vi "Logging Active.vi"(8 "error in (no error)":errorcluster, 11 "Active in":refnum<class "Active.lvclass">) -> (0 "error out":errorcluster, 3 "Active out":refnum<class "Active.lvclass">)   [LabVIEW 2024]
uses:
  Active.lvclass
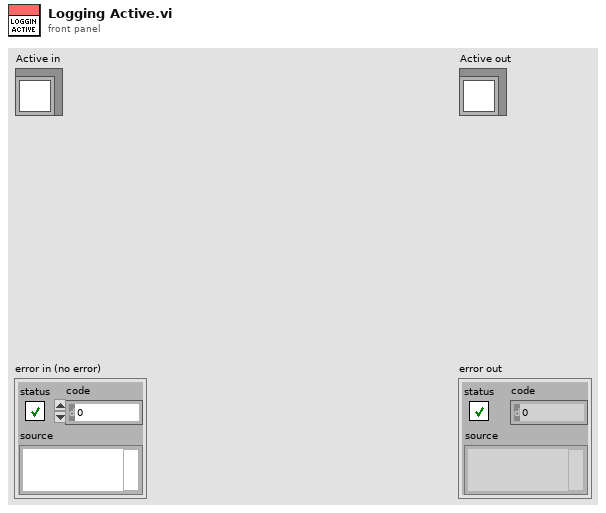
[diagram p1: front panel]
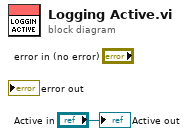
[diagram p0: block diagram]
diagram:
  "Active out" <- "Active in"
